vi "c ctre phoenixpro Request Control Position Torque Current FOC.vi"(4 "Slot":i32, 5 "FeedForward":dbl, 6 "Position":dbl, 7 "cancelOtherRequests":bool, 8 "error in (no error)":errorcluster, 9 "updateTime":dbl, 10 "ecuEncoding":u32, 11 "canbus":string) -> (0 "error out":errorcluster, 3 "function return":i32)   [LabVIEW 2020, in "CTRE_PhoenixTools.lvlib"]
doc: "CTREXPORT int c_ctre_phoenixpro_RequestControlPositionTorqueCurrentFOC(const char *canbus, uint32_t ecuEncoding, double updateTime, bool cancelOtherRequests, double Position, double FeedForward, int Slot);"
uses:
  CTRE_PhoenixTools.lvlib
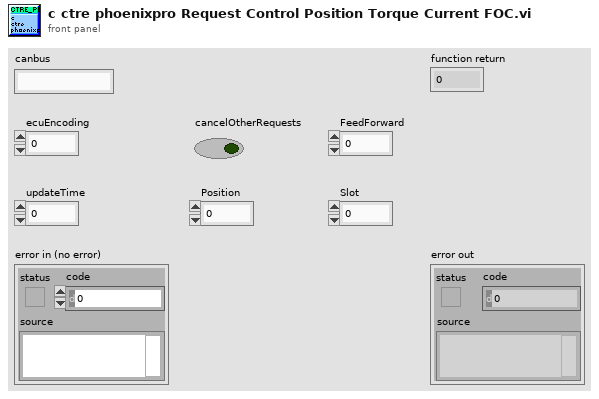
[diagram p1: front panel]
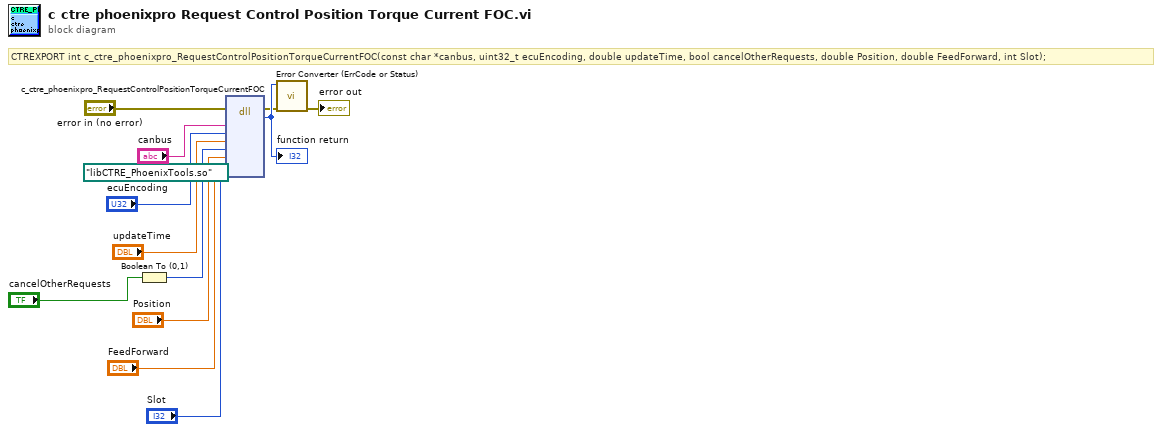
[diagram p0: block diagram]
diagram:
  # "CTREXPORT int c_ctre_phoenixpro_RequestControlPositionTorqueCurrentFOC(const char *canbus, uint32_t ecuEncoding, double updateTime, bool cancelOtherRequests, double Position, double FeedForward, int Slot);"
  n1 = Boolean To (0,1)(Boolean="cancelOtherRequests") -> (0, 1=w8:i16)
  n2 = dll-call lib="?" fn="c_ctre_phoenixpro_RequestControlPositionTorqueCurrentFOC"(path in=path "libCTRE_PhoenixTools.so", error in="error in (no error)", "canbus"="canbus", "ecuEncoding"="ecuEncoding", "updateTime"="updateTime", "cancelOtherRequests"=w8, "Position"="Position", "FeedForward"="FeedForward", "Slot"="Slot") -> (error out=w3:errorcluster, w13:i32)  [unwired: 8 in, 1 out]
  "function return" <- w13
  n3 = call "Error Converter (ErrCode or Status).vi"("error in (no error)"=w3, "error code"=w13) -> ("error out"=→"error out":errorcluster)  [unwired: 9 in]
